vi "FindUniqueAEs(SubVI).vi"(11 "Report DVR":refnum<data-value>) -> (3 "AE names array Out":string[](array[string]))   [LabVIEW 2018, in "DS_Lib.lvlib" / "SRReportParser.lvlib"]
uses:
  SRReportParser.lvlib
  Modules/Private Controls/Report Data Cluster.ctl
  Modules/Private Controls/Data Raw.ctl
  Modules/Data Operations.lvlib
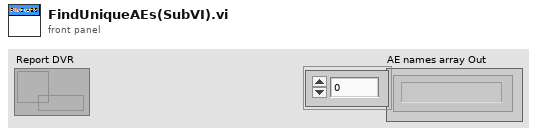
[diagram p1: front panel]
types:
  T1 = typedef "Data Operations.lvlib/Report Data Cluster.ctl" = cluster{"Headers":cluster{"Start Date":timestamp, "End Date":timestamp, "SR Status String":string[], "AE Owner String":string[]}, "Data":T2[]}
  T2 = typedef "Data Operations.lvlib/Data Raw.ctl" = cluster{"SR Number":string, "Status":string, "Summary":string, "AE Owner":string, "AE Group":string, "Contact":string, "SurveyData":cluster{"Resolution Time":dbl, "Total Satisfaction":dbl, "Response Time":dbl, "Courtesy":dbl, "Problem Solved":dbl, "Level of effort":dbl}, "Time Data":cluster{"Last Update Date":timestamp, "Creation Date":timestamp, "Creation week":i16, "Last Update Week":i16, "Creation Year":i16}}
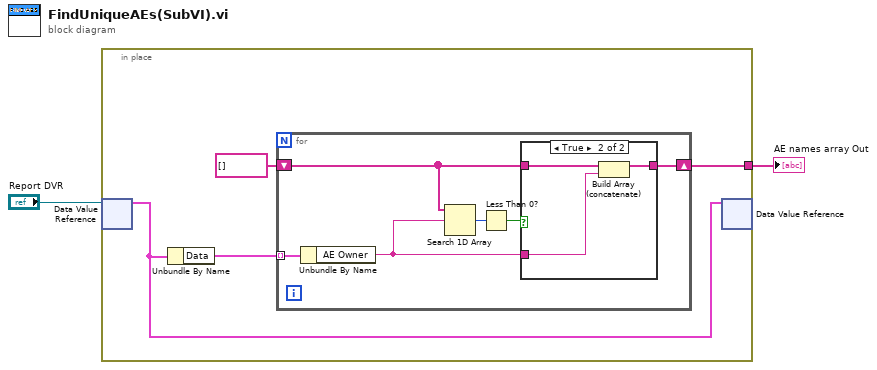
[diagram p0: block diagram]
diagram:
  n1 = in-place {
    in-place-border: [w6] -> w2
    n2 = in-place-dvr #1("Report DVR") -> (w3:T1)  [unwired: 1 out]
    n3 = Unbundle By Name(w3) -> ("Data"=w5:T2[])
    n4 = for {
      tunnel: w5 -> [w12] mode=indexing
      shift-right: [w8] -> w6
      shift-left: string[] [] -> [w7]
      n5 = Unbundle By Name(w12) -> ("AE Owner"=w9:string)
      n6 = Search 1D Array(1D array=w7, element=w9) -> (index of element=w11:i32)  [unwired: 1 in]
      n7 = Less Than 0?(x=w11) -> (x < 0?=w10:bool)
      n8 = case shown="True" w10 {
        tunnel: w9 -> [_ w14]
        tunnel: [w13 w16] -> w8
        tunnel: w7 -> [w13 w15]
        frame False {
        }
        frame True {
          n9 = Build Array (concatenate)(w15, w14) -> (w16:string[])
        }
      }
    }
    n10 = in-place-dvr #1(w3) -> ()  [unwired: 2 out]
  }
  "AE names array Out" <- w2
